vi "Update Setting.vi"(0 "Camera in":refnum<class "Camera.lvclass">, 1 "Setting":T1, 2 "Value":string, 3 "error in":errorcluster) -> (7 "Camera out":refnum<class "Camera.lvclass">, 8 "Supported?":bool, 10 "error out":errorcluster)   [LabVIEW 2018, in "Camera.lvlib" / "Camera.lvclass"]
uses:
  Camera.lvclass
  Custom Controls/Camera Setting.ctl
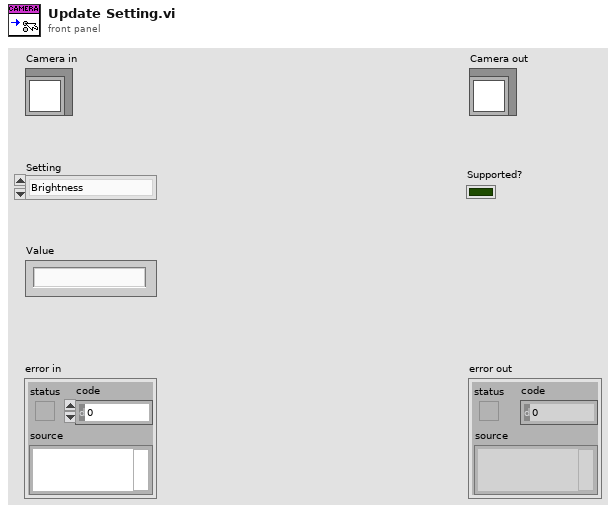
[diagram p1: front panel]
types:
  T1 = typedef "Camera.lvlib/Camera.lvclass/Camera Setting.ctl" = enum16{"Brightness", "Rotation", "Contrast", "Exposure", "Frame Rate", "Gain", "Gamma", "Image Resolution", "Sharpness"}
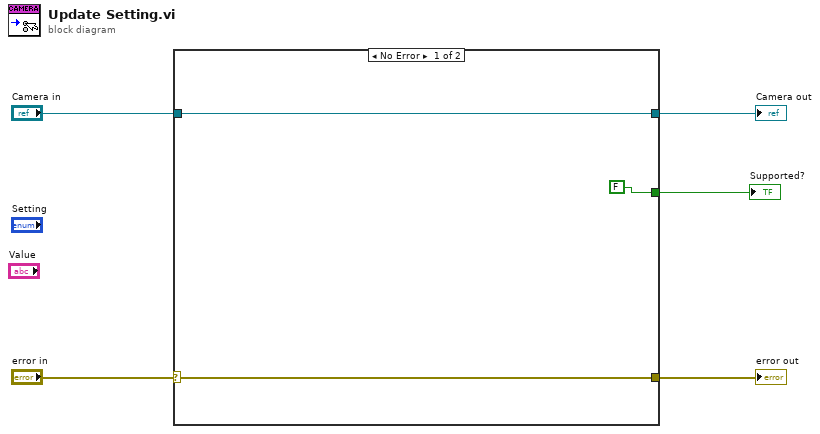
[diagram p0: block diagram]
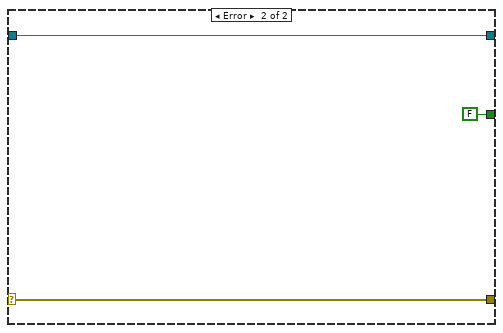
[diagram p2: hidden frame]
diagram:
  n1 = case shown="No Error" "error in" {
    selector: "error in" -> [w8 w10]
    tunnel: [w8 w10] -> w4
    tunnel: "Camera in" -> [w7 w11]
    tunnel: [w7 w11] -> w2
    tunnel: [FALSE FALSE] -> w1
    frame No Error {
    }
    frame Error {
    }
  }
  "error out" <- w4
  "Camera out" <- w2
  "Supported?" <- w1
